vi "006 Test SubVI Temp coherent.vi"() -> ()   [LabVIEW 2019]
panel:
  in  "Boolean":bool
  out "Min Temp":dbl
  out "Max Temp":dbl
  out "Alarma límit inf":bool
  out "Alarma límit sup":bool
  in  "Limit inferior":dbl
  in  "Limit superior":dbl
  out "Waveform Chart":T1(graph)
  out "Data":dbl
  in  "Conf. temperatura":T2
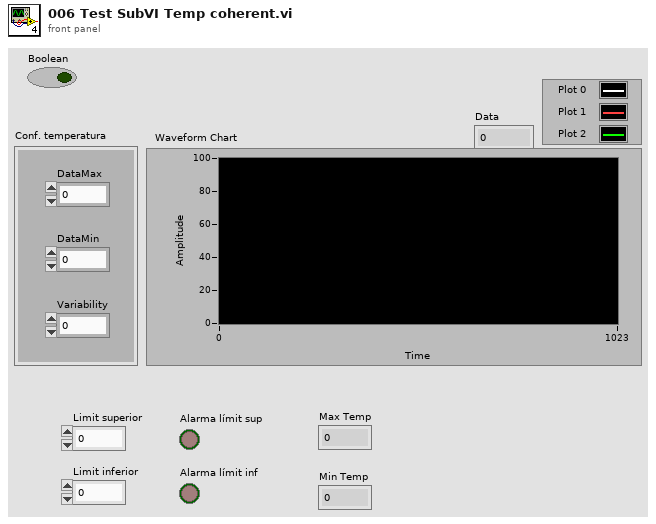
[diagram p1: front panel]
types:
  T1 = cluster{"Limit inferior":dbl, "Data":dbl, "Limit superior":dbl}
  T2 = cluster{"DataMin":dbl, "DataMax":dbl, "Variability":dbl}
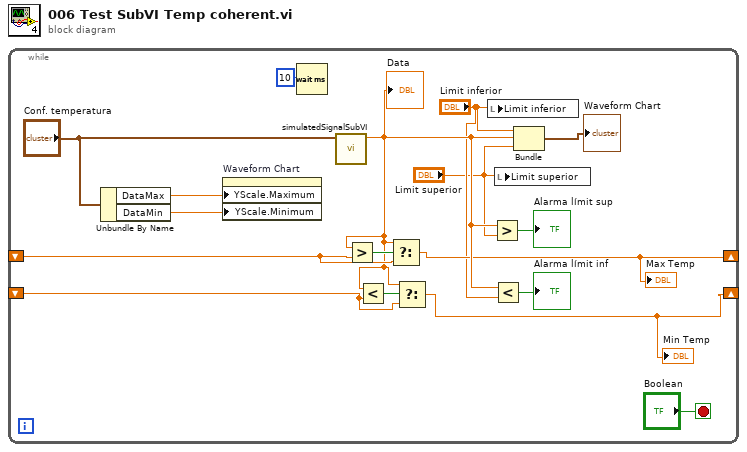
[diagram p0: block diagram]
diagram:
  n1 = while {
    shift-right: [w6] -> _
    shift-left: _ -> [w11]
    shift-right: [w7] -> _
    shift-left: _ -> [w8]
    stop <- "Boolean" stop-if-true
    n2 = Unbundle By Name("Conf. temperatura") -> ("DataMax"=w2:dbl, "DataMin"=w1:dbl)
    n3 = property on="Waveform Chart" class="WFChart (strict)"("YScale.Maximum"=w2, "YScale.Minimum"=w1) -> ()  [unwired: 2 in, 2 out]
    n4 = Wait (ms)(milliseconds to wait=u32 10) -> ()  [unwired: 1 out]
    n5 = call "simulatedSignalSubVI.vi"("Channel"="Conf. temperatura") -> ("Data"=w9:dbl)  [unwired: 10 in]
    "Data" <- w9
    n6 = Greater?(x=w9, y=w11) -> (0:w12:bool)
    n7 = Less?(x=w9, y=w8) -> (x < y?=w10:bool)
    n8 = Select(t=w9, s=w12, f=w11) -> (s? t:f=w6:dbl)
    "Max Temp" <- w6
    n9 = Select(t=w9, s=w10, f=w8) -> (s? t:f=w7:dbl)
    "Min Temp" <- w7
    n10 = local write "Limit inferior"("Limit inferior") -> ()
    n11 = Greater?(x=w9, y="Limit superior") -> (0:→"Alarma límit sup":bool)
    n12 = Less?(x=w9, y="Limit inferior") -> (x < y?=→"Alarma límit inf":bool)
    n13 = local write "Limit superior"("Limit superior") -> ()
    n14 = Bundle("Limit inferior"="Limit inferior", "Data"=w9, "Limit superior"="Limit superior") -> (→"Waveform Chart":T1)  [unwired: 1 in]
  }
